vi "basic - Receive Single Capture.vi"() -> ()   [LabVIEW 2020]
uses:
  src/AIM664LV.lvlib
  src/_polimorphicInstances/session/Fdx Create Session (RX-Monitor).vi
  src/_polimorphicInstances/control/Fdx Start (Rx).vi
  src/_polimorphicInstances/control/Fdx Stop (Rx).vi
  src/_polimorphicInstances/session/Fdx Close Session (Port).vi
  src/_controls/session_monitor_config.ctl
panel:
  in  "TriggerPosition":u32
  in  "Strobe":u32(ring) items=["FDX_MON_STROBE_DIS", "FDX_MON_STROBE_STOP", "FDX_MON_STROBE_START"]
  in  "CaptureMode":u32(ring) items=["FDX_MON_SINGLE ", "FDX_MON_CONTINUOUS", "FDX_MON_SELECTIVE", "FDX_MON_RECORDING", "FDX_MON_REROS", "FDX_MON_HMU"]
  in  "DefaultCronoMode":u32(ring)=2 items=["FDX_RX_DEFAULT_ENA_CNT", "FDX_RX_DEFAULT_MON_ENA_ALL", "FDX_RX_DEFAULT_MON_ENA_GOOD"]
  in  "Tab Control":enum32{"Package", "Statistics"}(tab)
  out "Synchronized":u32
  out "BytesRead":u32
  out "EntryRead":u32
  out "Data":string[][](table)
  out "Statistics":string[][](table)
  out "GlobalStat Out":T1
  in  "Control":u32(ring) items=["FDX_RX_GS_RES_NO_CNT", "FDX_RX_GS_RES_ALL_CNT", "FDX_RX_GS_RES_ERR_CNT"]
  in  "ReadQualifier (0:full)":u32
  in  "poll time ms":u32=100
  in  "QueueSize MB (1)":u32=1
  out "error out":errorcluster
  out "QueueStatus":T2 {"QueueStatus" items=["FDX_MON_STAT_EMPTY", "FDX_MON_STAT_ FILLED", "FDX_MON_STAT_ FULL", "FDX_MON_STAT_ OVERFLOW", "FDX_MON_STAT_ ERROR"]}
  out "GlobMonSize":u32
  out "PortInitOut":T3={"PortConfig"=0, "PortUsed"=1, "GlobalMemFree"=0, "SharedMemFree"=0} {"PortConfig" items=["FDX_SINGLE", "FDX_REDUNDANT"]}
  out "GlbMonBufferSizeOut":u32
  in  "board":u32
  in  "port":u32=1
  in  "DefaultPayloadMode (Full)":u32(ring) items=["FDX_PAYLOAD_FULL", "FDX_PAYLOAD_IP_EXT", "FDX_PAYLOAD_IP", "FDX_PAYLOAD_MAC"]
  in  "stop":bool
  out "current irig time":T4={"SignOut"=40, "DayOut"=1, "HourOut"=1, "MinOut"=28, "SecondOut"=39, "MilliSecOut"=539, "MicroSecOut"=300, "NanoSecOut"=0, "InfoOut"=0, "Mode"=3}
  out "current time":timestamp
  # "ARINC 664 Receive Continuous Capture"
  # "Overview: It helps to obtain the versions stored in the board.\n\nRequirement: One AIM ARINC-664 board with installed AIM ARINC 664 BSP.\nRestrictions: None.\nInstruction:\n1. Select the Board ID (0 if you have only one board in your system) and the port number. If you want to validate between two ports in one device, you can use tx board and Rx Boardd\n2. Run the VI.\n3. See the result in Current IRIG Time"
  # "Monitor Configuration"
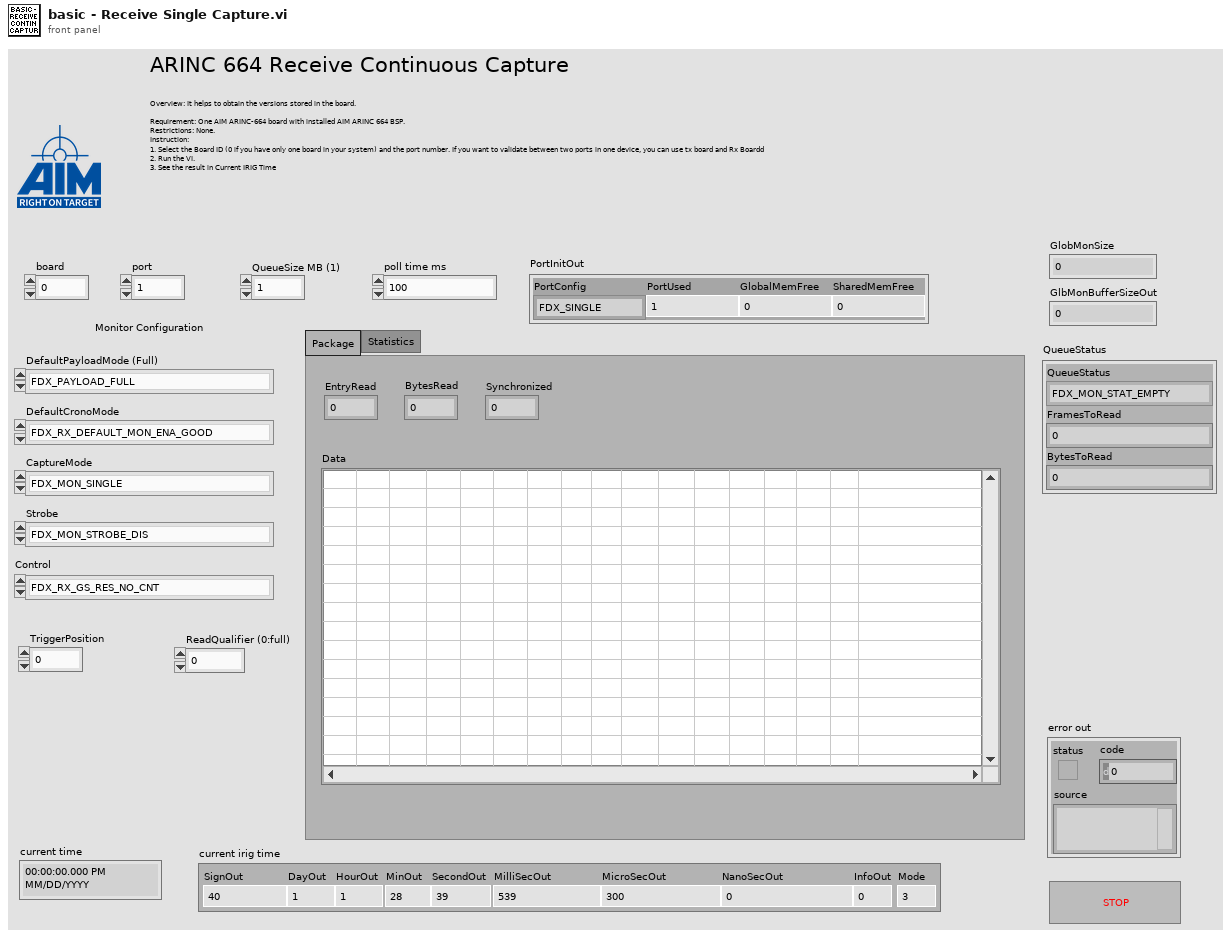
[diagram p1: front panel]
types:
  T1 = cluster{"TotalByteCount":u32[], "FrameGoodCount":u32[], "FrameErrorCount":u32[], "BytesPerSecond":u32[], "FramesPerSecond":u32[], "PhysErrorCount":u32[], "PreamErrorCount":u32[], "UnaligErrorCount":u32[], "CRCErrorCount":u32[], "IFGErrorCount":u32[], "IPErrorCount":u32[], "MACErrorCount":u32[], "NoSfdErrorCount":u32[], "VLLenErrorCount":u32[], "SNIntegrityErrorCount":u32[], "TrafShapingViolationCount":u32[], "MAC1Short":u32[], "MAC64To127Count":u32[], "MAC128To255Count":u32[], "MAC256To511Count":u32[], "MAC512To1023Count":u32[], "MAC1024To1518Count":u32[], "MACLong":u32[]}
  T2 = cluster{"QueueStatus":u32, "FramesToRead":u32, "BytesToRead":u32}
  T3 = cluster{"PortConfig":u32, "PortUsed":u32, "GlobalMemFree":u32, "SharedMemFree":u32}
  T4 = cluster{"SignOut":i32, "DayOut":u32, "HourOut":u32, "MinOut":u32, "SecondOut":u32, "MilliSecOut":u32, "MicroSecOut":u32, "NanoSecOut":u32, "InfoOut":u32, "Mode":u32}
  T5 = typedef "AIM664LV.lvlib/session_monitor_config.ctl" = cluster{"DefaultCronoMode":u32, "GlbMonBufferSizeIn":u32}
  T6 = cluster{"EntryRead":u32, "BytesRead":u32, "Synchronized":u32, "ReadBuffer":u8[]}
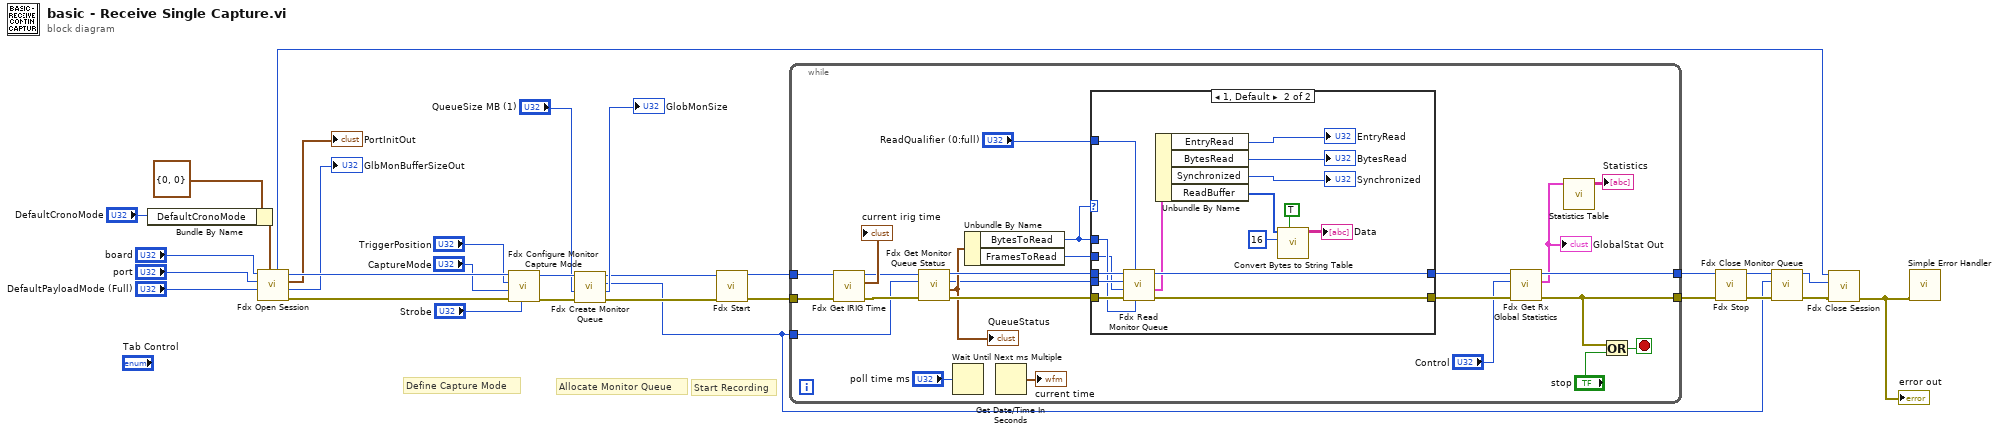
[diagram p0: block diagram]
diagram:
  # "Start Recording"
  # "Allocate Monitor Queue"
  # "Define Capture Mode"
  n1 = Bundle By Name(cluster=T5 {"DefaultCronoMode"=0, "GlbMonBufferSizeIn"=0} ("MonitorConfig"), "DefaultCronoMode"="DefaultCronoMode") -> (w5:T5)
  n2 = call-poly "Fdx Open Session.vi"("MonitorConfig"=w5, "DefaultPayloadMode (Full)"="DefaultPayloadMode (Full)", "port"="port", "board"="board") -> ("error out"=w29:errorcluster, "GlbMonBufferSizeOut"=→"GlbMonBufferSizeOut":u32, "PortInitOut"=→"PortInitOut":T3, "InstrumentHandle_port out"=w30:u32, "InstrumentHandle_board out"=w8:u32)  [unwired: 2 in, 1 out]
  n3 = call "Fdx Configure Monitor Capture Mode.vi"("Strobe"="Strobe", "error in (no error)"=w29, "CaptureMode"="CaptureMode", "TriggerPosition"="TriggerPosition", "InstrumentHandle_port in"=w30) -> ("error out"=w27:errorcluster, "InstrumentHandle_port out"=w28:u32)  [unwired: 5 in]
  n4 = call "Fdx Create Monitor Queue.vi"("error in (no error)"=w27, "MaxFileSize MB (1)"="QueueSize MB (1)", "InstrumentHandle_port in"=w28) -> ("error out"=w14:errorcluster, "GlobMonSize"=→"GlobMonSize":u32, "QueueIdOut"=w11:u32, "InstrumentHandle_port out"=w15:u32)  [unwired: 5 in]
  n5 = call-poly "Fdx Start.vi"("error in (no error)"=w14, "InstrumentHandle_port in"=w15) -> ("error out"=w20:errorcluster, "InstrumentHandle_port out"=w21:u32)  [unwired: 8 in]
  n6 = while {
    tunnel: [w36] -> w22
    tunnel: w21 -> [w49]
    tunnel: w20 -> [w48]
    tunnel: w11 -> [w42]
    tunnel: [w38] -> w16
    stop <- w53 stop-if-true
    n7 = call "Fdx Get IRIG Time.vi"("error in (no error)"=w48, "InstrumentHandle_board in"=w49) -> ("error out"=w47:errorcluster, "Curent Irig Time"=→"current irig time":T4, "InstrumentHandle_board out"=w43:u32)  [unwired: 7 in]
    n8 = call "Fdx Get Monitor Queue Status.vi"("error in (no error)"=w47, "QueueId in"=w42, "InstrumentHandle_port in"=w43) -> ("error out"=w46:errorcluster, "QueueStatus"=w44:T2, "QueueId out"=w41:u32, "InstrumentHandle_port out"=w45:u32)  [unwired: 5 in]
    "QueueStatus" <- w44
    n9 = Wait Until Next ms Multiple(millisecond multiple="poll time ms") -> ()  [unwired: 1 out]
    n10 = Unbundle By Name(w44) -> ("BytesToRead"=w33:u32, "FramesToRead"=w34:u32)
    n11 = Get Date/Time In Seconds() -> (seconds since 1Jan1904=→"current time":timestamp)
    n12 = case shown="1, Default" w33 {
      tunnel: w46 -> [w56 w72]
      tunnel: w45 -> [w55 w71]
      tunnel: w41 -> [_ w70]
      tunnel: [w55 w69] -> w40
      tunnel: [w56 w68] -> w39
      tunnel: w33 -> [_ w67]
      tunnel: "ReadQualifier (0:full)" -> [_ w66]
      tunnel: w34 -> [_ w65]
      frame 0 {
      }
      frame 1, Default {
        n13 = call "Fdx Read Monitor Queue.vi"("MaxReadBytes"=w67, "ReadQualifier (0:full)"=w66, "error in (no error)"=w72, "EntryCount (1)"=w65, "QueueId in"=w70, "InstrumentHandle_port in"=w71) -> ("error out"=w68:errorcluster, "QueueReadOut"=w64:T6, "InstrumentHandle_port out"=w69:u32)  [unwired: 2 in, 1 out]
        n14 = Unbundle By Name(w64) -> ("EntryRead"=→"EntryRead":u32, "BytesRead"=→"BytesRead":u32, "Synchronized"=→"Synchronized":u32, "ReadBuffer"=w61:u8[])
        n15 = call "Convert Bytes to String Table.vi"("Append ASCII Column?"=TRUE, "byters per row"=16, "Data"=w61) -> ("Data"=→"Data":string[][])  [unwired: 8 in]
      }
    }
    n16 = call "Fdx Get Rx Global Statistics.vi"("error in (no error)"=w39, "Control"="Control", "InstrumentHandle_port in"=w40) -> ("error out"=w38:errorcluster, "GlobalStat Out"=w32:T1, "InstrumentHandle_port out"=w36:u32)  [unwired: 6 in]
    "GlobalStat Out" <- w32
    n17 = call "Statistics Table.vi"("GlobalStat Out"=w32) -> ("Table Control"=→"Statistics":string[][])  [unwired: 10 in]
    n18 = Or(x=w38, y="stop") -> (x .or. y?=w53:bool)
  }
  n19 = call-poly "Fdx Stop.vi"("error in (no error)"=w16, "InstrumentHandle_port in"=w22) -> ("error out"=w18:errorcluster, "InstrumentHandle_port out"=w10:u32)  [unwired: 8 in]
  n20 = call "Fdx Close Monitor Queue.vi"("error in (no error)"=w18, "QueueId"=w11, "InstrumentHandle_port in"=w10) -> ("error out"=w17:errorcluster, "InstrumentHandle_port out"=w9:u32)  [unwired: 7 in]
  n21 = call-poly "Fdx Close Session.vi"("error in (no error)"=w17, "InstrumentHandle_port in"=w9, "InstrumentHandle_board in"=w8) -> ("error out"=w7:errorcluster)  [unwired: 8 in]
  "error out" <- w7
  n22 = call <vilib>:"Simple Error Handler.vi"("error in (no error)"=w7) -> ()  [unwired: 4 in, 5 out]
